vi "Run.vi"(8 "error in (no error)":errorcluster, 11 "Thread in":refnum<class "Thread.lvclass">) -> (0 "error out":errorcluster, 3 "Thread out":refnum<class "Thread.lvclass">)   [LabVIEW 2017, in "DSF Core.lvlib" / "Thread.lvclass"]
uses:
  Thread.lvclass
  Thread Command.ctl
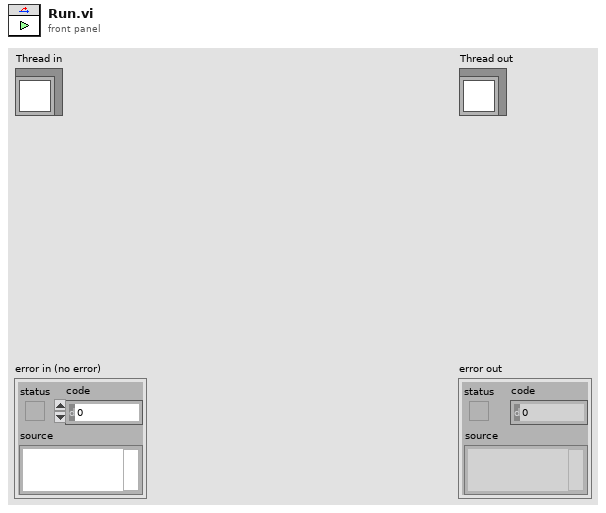
[diagram p1: front panel]
types:
  T1 = typedef "DSF Core.lvlib/Thread.lvclass/Thread State.ctl" = enum8{"Idle", "Running", "Error", "Shut Down"}
  T2 = typedef "DSF Core.lvlib/Thread.lvclass/Thread Command.ctl" = enum8{"Run", "Shutdown"}
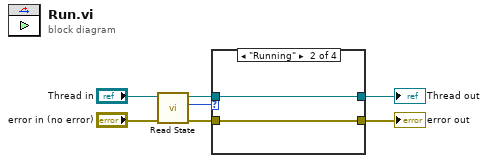
[diagram p0: block diagram]
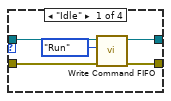
[diagram p2: hidden frame]
diagram:
  n1 = call "Read State.vi"("error in (no error)"="error in (no error)", "Thread in"="Thread in") -> ("error out"=w4:errorcluster, "state"=w3:T1, "Thread out"=w5:refnum<class "Thread.lvclass">)  [unwired: 7 in]
  n2 = case shown="\"Running\"" w3 {
    tunnel: w5 -> [w12 w14 w16 w17]
    tunnel: w4 -> [w11 w13 w15 w18]
    tunnel: [w10 w14 w16 w17] -> w1
    tunnel: [w9 w13 w15 w18] -> w2
    frame "Idle" {
      n3 = call "Write Command FIFO.vi"("error in (no error)"=w11, "command"=Thread_Command."Run", "Thread in"=w12) -> ("error out"=w9:errorcluster, "Thread out"=w10:refnum<class "Thread.lvclass">)  [unwired: 5 in, 2 out]
    }
    frame "Running" {
    }
    frame "Error" {
    }
    frame "Shut Down" {
    }
  }
  "error out" <- w2
  "Thread out" <- w1
